vi "Protokolldaten_leak check.vi"(0 "Daten":T1, 7 "Bearbeiter":string, 9 "Auswertung":string[](array[string]), 12 "Start":timestamp, 13 "Aktion":T2) -> (14 "Start":timestamp, 19 "Auswertung":string[](array[string]), 20 "Daten":T1, 27 "Bearbeiter":string)   [LabVIEW 2020, in "EPA 1065.lvlib" / "Dichtheitstest 1065-345.lvlib"]
uses:
  Dichtheitstest 1065-345.lvlib
  Aktion Protokolldaten_Leak check.ctl
  Leak Daten.ctl
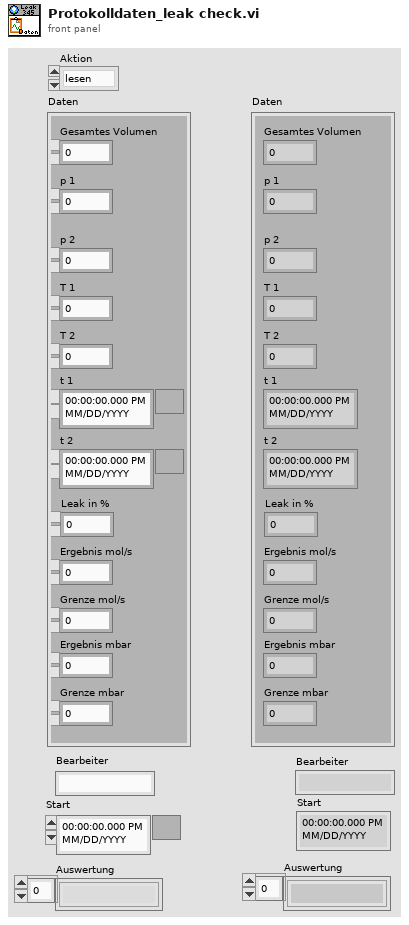
[diagram p1: front panel]
types:
  T1 = typedef "EPA 1065.lvlib/Dichtheitstest 1065-345.lvlib/Leak Daten.ctl" = cluster{"Gesamtes Volumen":sgl, "p 1":sgl, "p 2":sgl, "T 1":sgl, "T 2":sgl, "t 1":timestamp, "t 2":timestamp, "Ergebnis mol/s":sgl, "Grenze mol/s":sgl, "Leak in %":sgl, "Ergebnis mbar":sgl, "Grenze mbar":sgl}
  T2 = typedef "EPA 1065.lvlib/Dichtheitstest 1065-345.lvlib/Aktion Protokolldaten_Leak check.ctl" = enum16{"lesen", "Zeitstempel", "Bearbeiter", "Daten", "Auswertung", "löschen"}
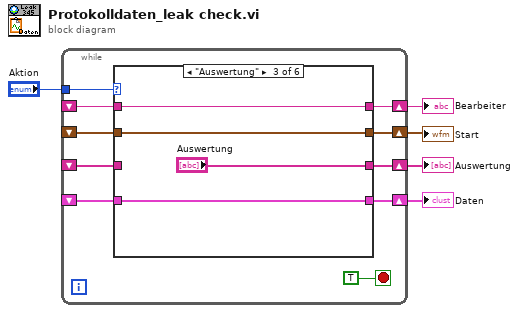
[diagram p0: block diagram]
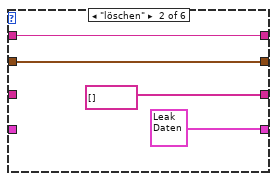
[diagram p3: hidden frame]
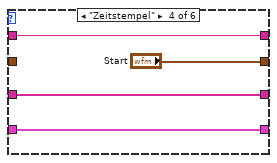
[diagram p4: hidden frame]
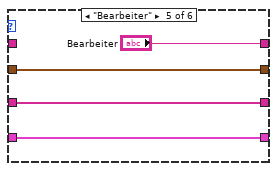
[diagram p5: hidden frame]
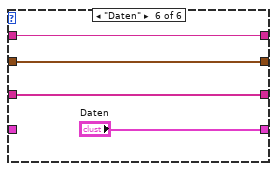
[diagram p6: hidden frame]
diagram:
  n1 = while {
    tunnel: "Aktion" -> [w14]
    shift-right: [w13] -> w3
    shift-left: _ -> [w12]
    shift-right: [w11] -> w4
    shift-left: _ -> [w10]
    shift-right: [w9] -> w2
    shift-left: _ -> [w8]
    shift-right: [w7] -> w1
    shift-left: _ -> [w6]
    stop <- TRUE stop-if-true
    n2 = case shown="\"Auswertung\"" w14 {
      tunnel: [w19 w23 w27 "Start" w35 w39] -> w13
      tunnel: w12 -> [w19 w23 w27 _ w35 w39]
      tunnel: [w18 w22 w26 w30 "Bearbeiter" w38] -> w11
      tunnel: w10 -> [w18 w22 w26 w30 _ w38]
      tunnel: [w17 string[] [] ("Auswertung") "Auswertung" w29 w33 w37] -> w9
      tunnel: w8 -> [w17 _ _ w29 w33 w37]
      tunnel: [w16 T1 {"Gesamtes Volumen"=0.0, "p 1"=0.0, "p 2"=0.0, "T 1"=0.0, "T 2"=0.0, "t 1"=timestamp(0 s since 1904-01-01), "t 2"=timestamp(0 s since 1904-01-01), "Ergebnis mol/s"=0.0, "Grenze mol/s"=0.0, "Leak in %"=0.0, "Ergebnis mbar"=0.0, "Grenze mbar"=0.0} ("Daten") w24 w28 w32 "Daten"] -> w7
      tunnel: w6 -> [w16 _ w24 w28 w32 _]
      frame "lesen", Default {
      }
      frame "löschen" {
      }
      frame "Auswertung" {
      }
      frame "Zeitstempel" {
      }
      frame "Bearbeiter" {
      }
      frame "Daten" {
      }
    }
  }
  "Bearbeiter" <- w4
  "Start" <- w3
  "Auswertung" <- w2
  "Daten" <- w1
